vi "Greater or Equal with Epsilon.vi"(10 "b":dbl, 11 "a":dbl) -> (3 "a>=b":bool)   [LabVIEW 2018, in "Waveform Equalizer.lvlib"]
uses:
  Waveform Equalizer.lvlib
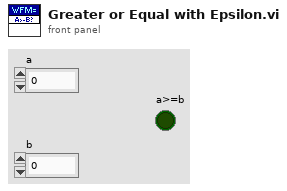
[diagram p1: front panel]
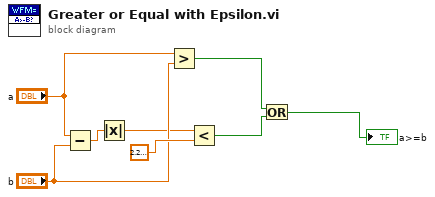
[diagram p0: block diagram]
diagram:
  n1 = Subtract(x="a", y="b") -> (x-y=w8:dbl)
  n2 = Absolute Value(x=w8) -> (abs(x)=w1:dbl)
  n3 = Greater?(x="a", y="b") -> (0:w3:bool)
  n4 = Less?(x=w1, y=2.220446049250313e-16) -> (x < y?=w4:bool)
  n5 = Or(x=w3, y=w4) -> (x .or. y?=→"a>=b":bool)
